vi "Add Message Error.vi"(9 "create message error":bool, 10 "Message in":T1) -> (2 "Message out":T1)   [LabVIEW 2019, in "RemoteControl.lvlib" / "RemoteControl.lvclass"]
uses:
  RemoteControl.lvclass
  Typedefs/Message--Cluster.ctl
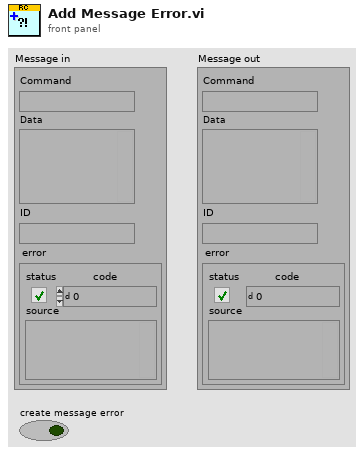
[diagram p1: front panel]
types:
  T1 = typedef "RemoteControl.lvlib/RemoteControl.lvclass/Message--Cluster.ctl" = cluster{"Command":string, "Data":variant, "ID":string, "error":errorcluster}
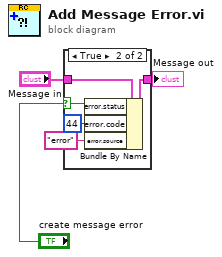
[diagram p0: block diagram]
diagram:
  n1 = case shown="True" "create message error" {
    selector: "create message error" -> [_ w7]
    tunnel: "Message in" -> [w4 w9]
    tunnel: [w4 w8] -> w2
    frame False {
    }
    frame True {
      n2 = Bundle By Name(cluster=w9, "error.status"=w7, "error.code"=44, "error.source"="error") -> (w8:T1)
    }
  }
  "Message out" <- w2
